vi "Create Dual Tone Signal.vi"(8 "error in (no error)":errorcluster, 10 "number of channels":u32=1, 11 "dual tone properties":T1) -> (0 "error out":errorcluster, 3 "signals":refnum<class "SV Multitone.lvclass">[](array[class]))   [LabVIEW 2021, in "AnalogGenerationProcess.lvlib"]
uses:
  AnalogGenerationProcess.lvlib
  <vilib>/addons/_NISVFA/_Generation/Signal Generation/SV Multitone/SV Multitone.lvclass
  controls/dual tone properties.ctl
  controls/dual tone types.ctl
  <vilib>/addons/_NISVFA/_Generation/Signal Generation/SV Multitone/Configure Multitone (Custom).vi
  <vilib>/addons/_NISVFA/_Generation/Signal Generation/SV Signal/SV Signal.lvclass
  controls/AudioGenTypeDefs.lvlib
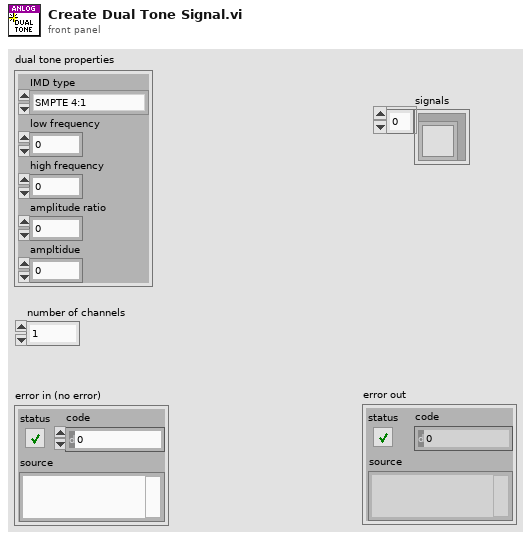
[diagram p1: front panel]
types:
  T1 = typedef "AudioGenTypeDefs.lvlib/dual tone properties.ctl" = cluster{"IMD type":T2, "low frequency":dbl, "high frequency":dbl, "amplitude ratio":dbl, "ampltidue":dbl}
  T2 = typedef "AudioGenTypeDefs.lvlib/dual tone types.ctl" = enum32{"SMPTE 4:1", "DIN", "CCIF 11k-12k", "CCIF 19k-20k", "Custom"}
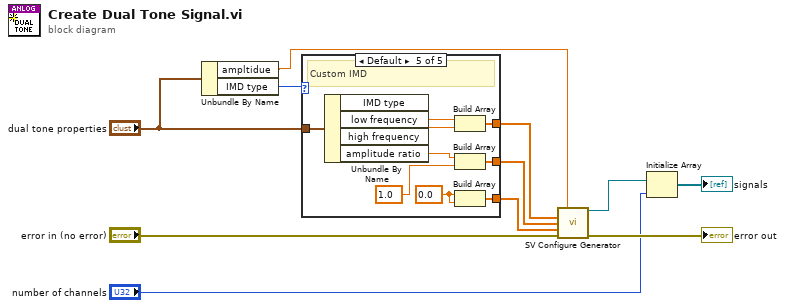
[diagram p0: block diagram]
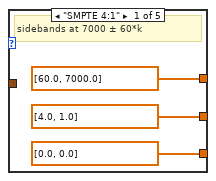
[diagram p2: hidden frame]
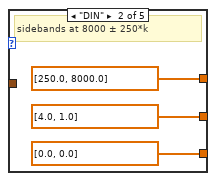
[diagram p3: hidden frame]
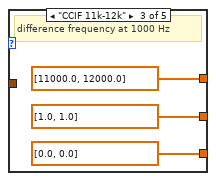
[diagram p4: hidden frame]
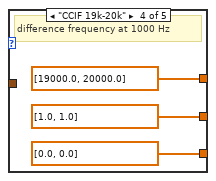
[diagram p5: hidden frame]
diagram:
  n1 = Unbundle By Name("dual tone properties") -> ("ampltidue"=w1:dbl, "IMD type"=w5:T2)
  n2 = case shown="Default" w5 {
    tunnel: [dbl[] [60.0, 7000.0] ("source settings.frequencies") dbl[] [250.0, 8000.0] ("source settings.frequencies") dbl[] [11000.0, 12000.0] ("source settings.frequencies") dbl[] [19000.0, 20000.0] ("source settings.frequencies") w26] -> w9
    tunnel: [dbl[] [4.0, 1.0] ("source settings.frequencies") dbl[] [4.0, 1.0] ("source settings.frequencies") dbl[] [1.0, 1.0] ("source settings.frequencies") dbl[] [1.0, 1.0] ("source settings.frequencies") w32] -> w8
    tunnel: [dbl[] [0.0, 0.0] ("source settings.frequencies") dbl[] [0.0, 0.0] ("source settings.frequencies") dbl[] [0.0, 0.0] ("source settings.frequencies") dbl[] [0.0, 0.0] ("source settings.frequencies") w27] -> w7
    tunnel: "dual tone properties" -> [_ _ _ _ w24]
    frame "SMPTE 4:1" {
      # "sidebands at 7000 ± 60*k"
    }
    frame "DIN" {
      # "sidebands at 8000 ± 250*k"
    }
    frame "CCIF 11k-12k" {
      # "difference frequency at 1000 Hz"
    }
    frame "CCIF 19k-20k" {
      # "difference frequency at 1000 Hz"
    }
    frame Default {
      w28 = 0.0 ("element")
      # "Custom IMD"
      n3 = Unbundle By Name(w24) -> ("low frequency"=w30:dbl, "high frequency"=w31:dbl, "amplitude ratio"=w25:dbl)  [unwired: 1 out]
      n4 = Build Array(w30, w31) -> (w26:dbl[])
      n5 = Build Array(w25, 1.0 ("element")) -> (w32:dbl[])
      n6 = Build Array(w28, w28) -> (w27:dbl[])
    }
  }
  n7 = call-poly <vilib>:"SV Configure Generator.vi"("overall amplitude"=w1, "frequencies [Hz]"=w9, "amplitudes"=w8, "phases [deg]"=w7, "error in (no error)"="error in (no error)") -> ("signal configuration"=w4:refnum<class "SV Multitone.lvclass">, "error out"=→"error out":errorcluster)  [unwired: 8 in, 1 out]
  n8 = Initialize Array(w4, "number of channels") -> (→"signals":refnum<class "SV Multitone.lvclass">[])
